vi "RSZVB Set Signal Source.vi"(6 "Port Number (1)":i32=1, 7 "Source (Port)":i32(ring)=1 items=["None", "Port", "Generator", "Embeded"], 8 "error in (no error)":errorcluster {"code" format="%.0x"}, 9 "Stage (1)":i32=1, 10 "Channel (1)":i32=1, 11 "VISA resource name":refnum<visa-resource-name>) -> (0 "error out":errorcluster {"code" format="%.0x"}, 3 "VISA resource name out":refnum<visa-resource-name>)   [LabVIEW 2011]
doc: "This VI selects an analyzer or an external generator port as a signal source for the LO 1 or L0 2 signal.\n\nNotes:\n\n(1) For mixer delay measurements and vector mixer measurements (options R&S ZVA-K5, R&S ZVAK9, R&S ZVA-K10), ports 1 and 2 are reserved for the RF and IF signals, respectively. Only a\nsingle mixer stage (<Stg> = 1) is supported.\n\nRemote-control command(s):\n[SENSe<Ch>:]FREQuency:CONVersion:MIXer:LOPort<Stg> NONE | EMBedded | PORT, <port_number> | GENerator, <gen_number>"
uses:
  _utility/RSZVB Global Data.vi
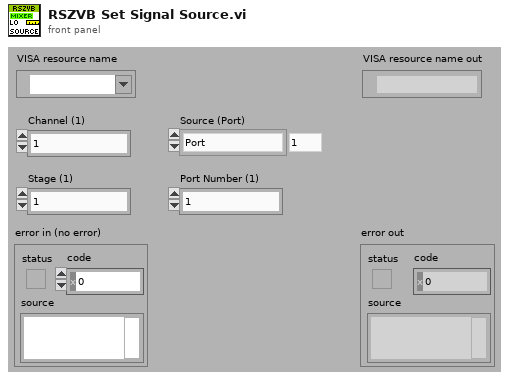
[diagram p1: front panel]
types:
  T1 = cluster{"Error Checking (T: On)":bool, "Installed Options":string[], "Data Valid?":bool, "Ports":i32, "Model":string[], "Option Checking (T: On)":bool}[]
  T2 = cluster{"Error Checking (T: On)":bool, "Installed Options":string[], "Data Valid?":bool, "Ports":i32, "Model":string[], "Option Checking (T: On)":bool}
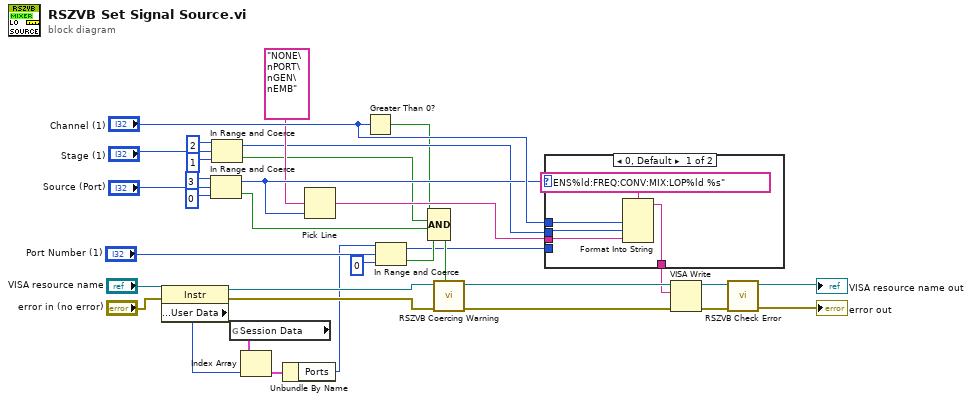
[diagram p0: block diagram]
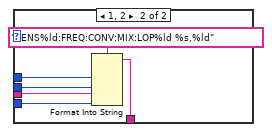
[diagram p2: hidden frame]
diagram:
  n1 = property class="Instr"(reference="VISA resource name", error in="error in (no error)") -> (reference out=w20:refnum<visa-resource-name>, error out=w21:errorcluster, "General Settings:User Data"=w24:u32)
  n2 = In Range and Coerce(upper limit=3, x="Source (Port)", lower limit=0) -> (coerced(x)=w10:i32, In Range?=w3:bool)
  n3 = In Range and Coerce(upper limit=2, x="Stage (1)", lower limit=1) -> (coerced(x)=w7:i32, In Range?=w4:bool)
  n4 = global read "RSZVB Global Data.vi" "Session Data"() -> (w25:T1)
  n5 = Index Array(array=w25, index=w24) -> (element=w26:T2)
  n6 = Unbundle By Name(w26) -> ("Ports"=w12:i32)
  n7 = Pick Line(multi-line string="NONE\nPORT\nGEN\nEMB", line index=w10) -> (output string=w8:string)  [unwired: 1 in]
  n8 = Greater Than 0?(x="Channel (1)") -> (x > 0?=w6:bool)
  n9 = In Range and Coerce(upper limit=w12, x="Port Number (1)", lower limit=0) -> (coerced(x)=w2:i32, In Range?=w5:bool)
  n10 = Compound Arithmetic op=AND(w6, w4, w3, w5) -> (w29:bool)
  n11 = call "RSZVB Coercing Warning.vi"("In Range?"=w29, "error in (no error)"=w21, "VISA session"=w20) -> ("error out"=w32:errorcluster, "dup VISA session"=w33:refnum<visa-resource-name>)  [unwired: 7 in]
  n12 = case shown="0, Default" w10 {
    tunnel: "Channel (1)" -> [w37 w43]
    tunnel: w8 -> [w36 w41]
    tunnel: w7 -> [w35 w42]
    tunnel: w2 -> [_ w40]
    tunnel: [w38 w44] -> w1
    frame 0, Default {
      n13 = Format Into String(format string="SENS%ld:FREQ:CONV:MIX:LOP%ld %s", w37, w35, w36) -> (resulting string=w38:string)  [unwired: 2 in, 1 out]
    }
    frame 1, 2 {
      n14 = Format Into String(format string="SENS%ld:FREQ:CONV:MIX:LOP%ld %s,%ld", w43, w42, w41, w40) -> (resulting string=w44:string)  [unwired: 2 in, 1 out]
    }
  }
  n15 = VISA Write(VISA resource name=w33, write buffer=w1, error in (no error)=w32) -> (VISA resource name out=w30:refnum<visa-resource-name>, error out=w31:errorcluster)  [unwired: 1 out]
  n16 = call "RSZVB Check Error.vi"("error in (no error)"=w31, "VISA session"=w30) -> ("error out"=→"error out":errorcluster, "dup VISA session"=→"VISA resource name out":refnum<visa-resource-name>)  [unwired: 8 in]
